vi "Close.vi"(8 "error in (no error)":errorcluster, 11 "handle in":u32) -> (0 "error out":errorcluster)   [LabVIEW 2016, in "Drivers.lvlib" / "C8855-01.lvlib"]
doc: "Releases the handle obtained with Open or MOpen.\n\n\n\nBOOL C8855API __stdcall C8855Close( HANDLE hC8855 );"
uses:
  C8855-01.lvlib
  C8855-01api.dll
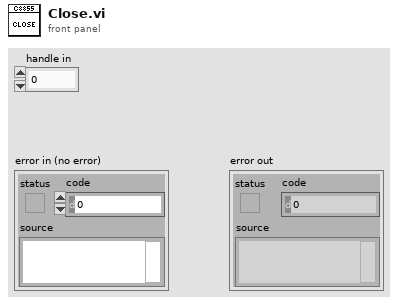
[diagram p1: front panel]
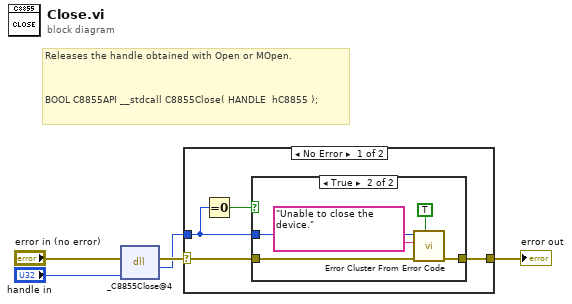
[diagram p0: block diagram]
diagram:
  # "Releases the handle obtained with Open or MOpen.\n\n\n\nBOOL C8855API __stdcall C8855Close( HANDLE  hC8855 );"
  n1 = dll-call lib="Z:/TraceGrabber/Drivers/C8855-01/C8855-01api.*" fn="_C8855Close@4"(error in="error in (no error)", "Handle"="handle in") -> (error out=w3:errorcluster, w2:i32)  [unwired: 3 in, 1 out]
  n2 = case shown="No Error" w3 {
    selector: w3 -> [w8 w16]
    tunnel: w2 -> [w6 _]
    tunnel: [w7 w16] -> w1
    frame No Error {
      n3 = Equal To 0?(x=w6) -> (x = 0?=w9:bool)
      n4 = case shown="True" w9 {
        tunnel: w8 -> [w10 w14]
        tunnel: [w10 w13] -> w7
        tunnel: w6 -> [_ w12]
        frame False {
        }
        frame True {
          n5 = call <vilib>:"Error Cluster From Error Code.vi"("show call chain? (False)"=TRUE, "error in (no error)"=w14, "error message (\"\")"="Unable to close the device." ("error message (\"\")"), "error code (0)"=w12) -> ("error out"=w13:errorcluster)  [unwired: 5 in]
        }
      }
    }
    frame Error {
    }
  }
  "error out" <- w1
